vi "Back Out Current Page Hierarchy.vi"(8 "error in (no error)":errorcluster, 11 "VIDoc Printer - Confluence In":refnum<class "VIDoc Printer - Confluence.lvclass">) -> (0 "error out":errorcluster, 3 "VIDoc Printer - Confluence Out":refnum<class "VIDoc Printer - Confluence.lvclass">)   [LabVIEW 2023, in "VIDoc Printer - Confluence.lvlib" / "VIDoc Printer - Confluence.lvclass"]
uses:
  VIDoc Printer - Confluence.lvclass
  VIDoc Printer - Confluence.lvclass/VIDoc Printer - Confluence.ctl
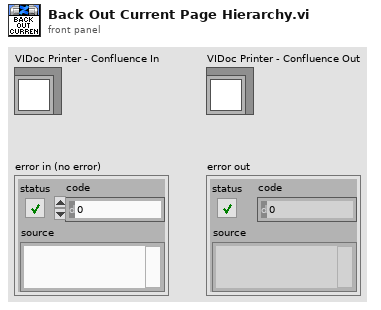
[diagram p1: front panel]
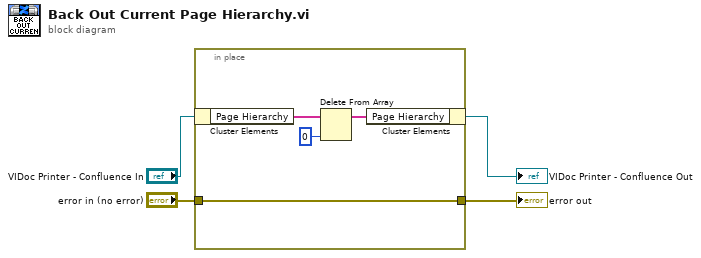
[diagram p0: block diagram]
diagram:
  n1 = in-place {
    in-place-border: [w5] -> w3
    in-place-border: "error in (no error)" -> [w5]
    n2 = in-place-cluster #1("VIDoc Printer - Confluence In") -> ("Page Hierarchy"=w8:string[])
    n3 = Delete From Array(array=w8, index=0) -> (array with subset deleted=w7:string[])  [unwired: 1 in, 1 out]
    n4 = in-place-cluster #1("Page Hierarchy"=w7) -> (→"VIDoc Printer - Confluence Out":refnum<class "VIDoc Printer - Confluence.lvclass">)
  }
  "error out" <- w3
